vi "Signal_buffer.vi"(0 "Queue in":refnum<queue>, 1 "Bufer1 IN":dbl[](array[numeric]), 2 "Buffer0 IN":dbl[](array[numeric]), 3 "SYSTEM SETTINGS":T2, 4 "Input controls (cluster)":T1={"TIME OFFSET 1"=1000000, "OFFSET UNIT"="", "TIME OFFSET 0"=1000000, "OFFSET UNIT 2"="", "OFFSET 0"=0.0, "OFFSET 1"=0.0} {"TIME OFFSET 0" scale=100000.0..1000000.0; "TIME OFFSET 1" scale=100000.0..1000000.0}, 5 "error in (no error)":errorcluster) -> (14 "Queue out":refnum<queue>, 15 "Waveform 1":waveform(dbl), 16 "Buffer1 OUT":dbl[](array[numeric]), 17 "Buffer0 OUT":dbl[](array[numeric]), 18 "Waveform 0":waveform(dbl), 19 "error out":errorcluster)   [LabVIEW 2019]
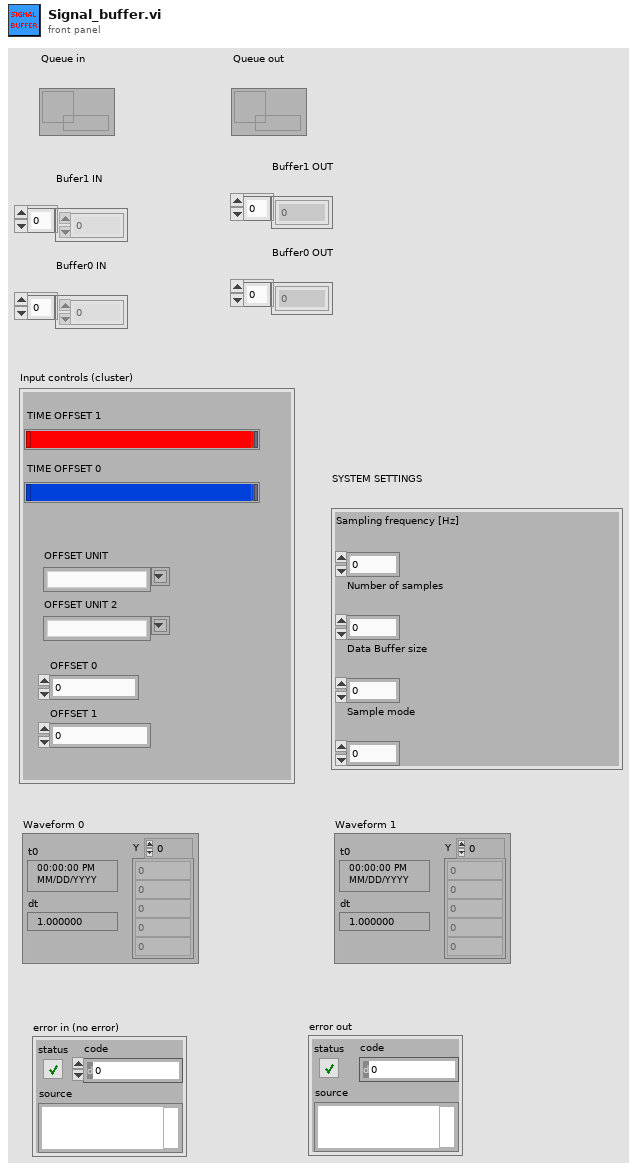
[diagram p1: front panel]
types:
  T1 = cluster{"TIME OFFSET 1":i32, "OFFSET UNIT":string, "TIME OFFSET 0":i32, "OFFSET UNIT 2":string, "OFFSET 0":dbl, "OFFSET 1":dbl}
  T2 = cluster{"Sampling frequency [Hz]":dbl, "Number of samples":i32, "Data Buffer size":i32, "Sample mode":i32}
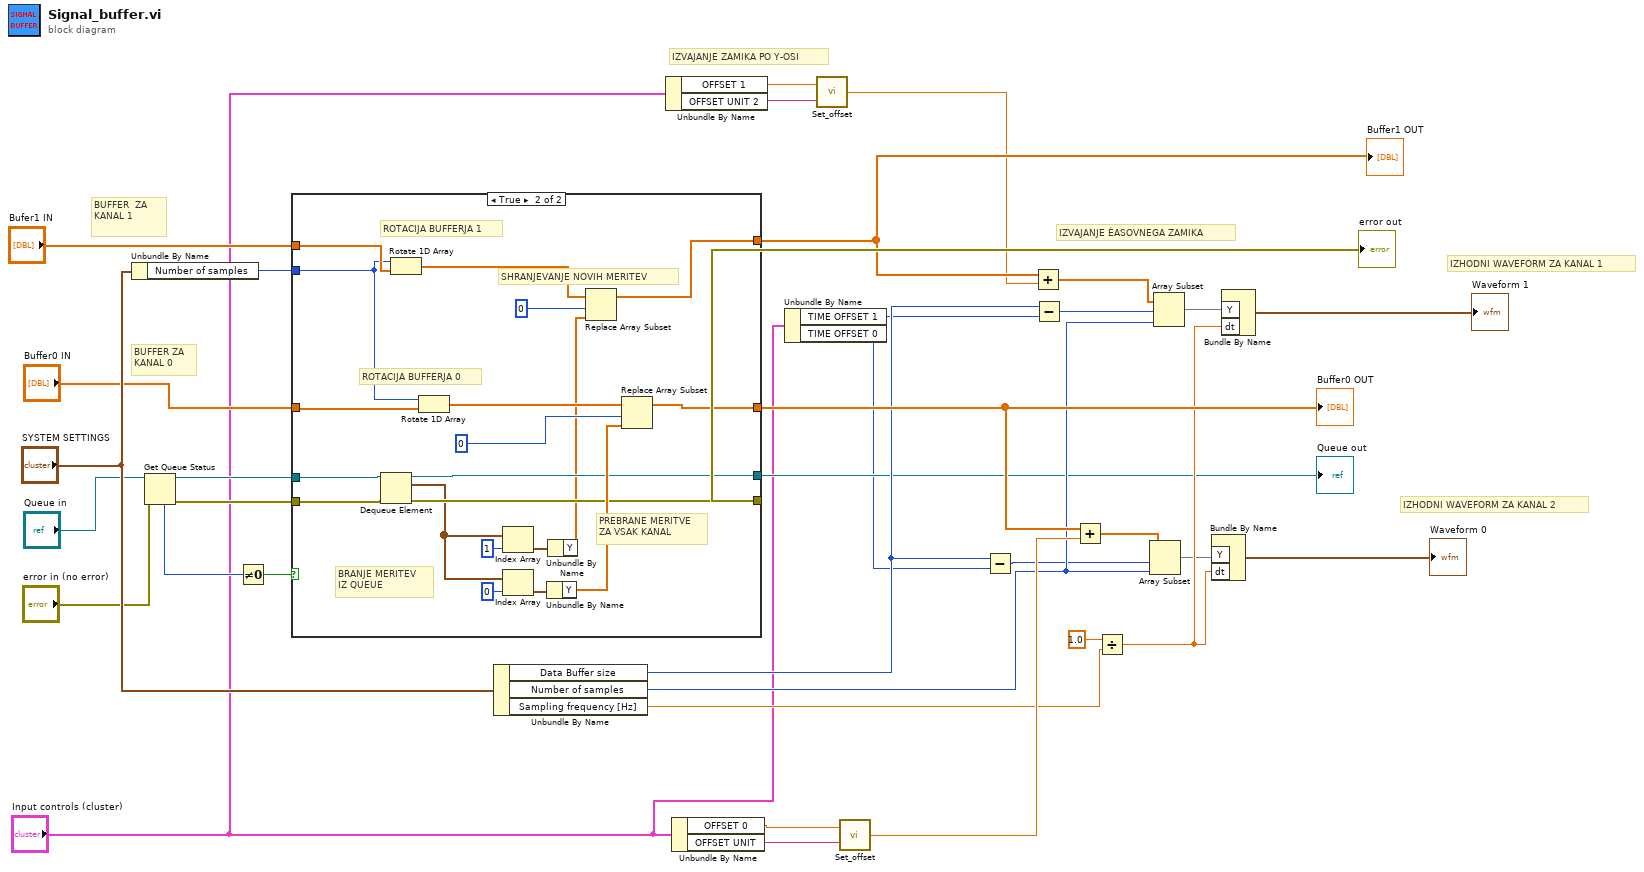
[diagram p0: block diagram]
diagram:
  # "IZHODNI WAVEFORM ZA KANAL 2"
  # "BUFFER ZA \nKANAL 0"
  # "IZVAJANJE ZAMIKA PO Y-OSI"
  # "IZHODNI WAVEFORM ZA KANAL 1"
  # "IZVAJANJE ÈASOVNEGA ZAMIKA"
  # "BUFFER  ZA KANAL 1"
  n1 = Unbundle By Name("SYSTEM SETTINGS") -> ("Number of samples"=w17:i32)
  n2 = Get Queue Status(queue="Queue in", error in (no error)="error in (no error)") -> (queue out=w13:refnum<queue>, error out=w12:errorcluster, # elements in queue=w11:i32)  [unwired: 1 in, 5 out]
  n3 = Not Equal To 0?(x=w11) -> (x != 0?=w10:bool)
  n4 = case shown="True" w10 {
    tunnel: w12 -> [w38 w59]
    tunnel: w13 -> [w39 w60]
    tunnel: "Buffer0 IN" -> [w40 w58]
    tunnel: [w40 w55] -> w33
    tunnel: w17 -> [_ w41]
    tunnel: [w39 w53] -> w20
    tunnel: [w38 w52] -> w35
    tunnel: "Bufer1 IN" -> [w37 w49]
    tunnel: [w37 w47] -> w30
    frame False {
    }
    frame True {
      # "ROTACIJA BUFFERJA 0"
      # "PREBRANE MERITVE\nZA VSAK KANAL"
      # "BRANJE MERITEV \nIZ QUEUE"
      # "SHRANJEVANJE NOVIH MERITEV"
      # "ROTACIJA BUFFERJA 1"
      n5 = Dequeue Element(queue=w60, error in (no error)=w59) -> (queue out=w53:refnum<queue>, element=w44:waveform(dbl)[], error out=w52:errorcluster)  [unwired: 1 in, 1 out]
      n6 = Rotate 1D Array(1:w49, 2:w41) -> (0:w48:dbl[])
      n7 = Rotate 1D Array(1:w58, 2:w41) -> (0:w57:dbl[])
      n8 = Index Array(array=w44, index=1) -> (element=w43:waveform(dbl))
      n9 = Index Array(array=w44, index=0) -> (element=w50:waveform(dbl))
      n10 = Unbundle By Name(w50) -> ("Y"=w54:dbl[])
      n11 = Unbundle By Name(w43) -> ("Y"=w42:dbl[])
      n12 = Replace Array Subset(array=w48, new element=w42, index=0) -> (w47:dbl[])
      n13 = Replace Array Subset(array=w57, new element=w54, index=0) -> (w55:dbl[])
    }
  }
  "error out" <- w35
  "Buffer0 OUT" <- w33
  "Buffer1 OUT" <- w30
  "Queue out" <- w20
  n14 = Unbundle By Name("SYSTEM SETTINGS") -> ("Data Buffer size"=w25:i32, "Number of samples"=w26:i32, "Sampling frequency [Hz]"=w19:dbl)
  n15 = Unbundle By Name("Input controls (cluster)") -> ("OFFSET 1"=w4:dbl, "OFFSET UNIT 2"=w5:string)
  n16 = Unbundle By Name("Input controls (cluster)") -> ("OFFSET 0"=w6:dbl, "OFFSET UNIT"=w7:string)
  n17 = Unbundle By Name("Input controls (cluster)") -> ("TIME OFFSET 1"=w2:i32, "TIME OFFSET 0"=w3:i32)
  n18 = call "Set_offset.vi"("OFFSET UNIT"=w5, "OFFSET VALUE in"=w4) -> ("OFFSET VALUE out"=w28:dbl)
  n19 = call "Set_offset.vi"("OFFSET UNIT"=w7, "OFFSET VALUE in"=w6) -> ("OFFSET VALUE out"=w32:dbl)
  n20 = Subtract(x=w25, y=w3) -> (x-y=w23:i32)
  n21 = Add(x=w30, y=w28) -> (x+y=w29:dbl[])
  n22 = Subtract(x=w25, y=w2) -> (x-y=w24:i32)
  n23 = Add(x=w33, y=w32) -> (x+y=w31:dbl[])
  n24 = Divide(x=1.0, y=w19) -> (x/y=w27:dbl)
  n25 = Array Subset(array=w31, index=w23, length=w26) -> (w15:dbl[])
  n26 = Array Subset(array=w29, index=w24, length=w26) -> (w22:dbl[])
  n27 = Bundle By Name("Y"=w15, "dt"=w27) -> (→"Waveform 0":waveform(dbl))  [unwired: 1 in]
  n28 = Bundle By Name("Y"=w22, "dt"=w27) -> (→"Waveform 1":waveform(dbl))  [unwired: 1 in]
